vi "Get Job Data.vi"(0 "SystemLink repo in":T3, 5 "job ID":string, 11 "error in (no error)":errorcluster) -> (4 "SystemLink repo out":T3, 6 "job data":T1, 15 "error out":errorcluster)   [LabVIEW 2017, in "SystemLink_Repo_API.lvlib"]
doc: "Returns the job data for the specified job ID."
uses:
  SystemLink_Repo_API.lvlib
  systemlink repo.ctl
  <vilib>/httpClient/ClientHandle.ctl
  syslink_job.ctl
  syslink_job_datatype.ctl
  <vilib>/httpClient/LabVIEWHTTPClient.lvlib
panel:
  out "body":string
  out "headers":string
  # "Status will be \"SUCCEEDED\" for a successful job and \"FAILED\" for a failed job."
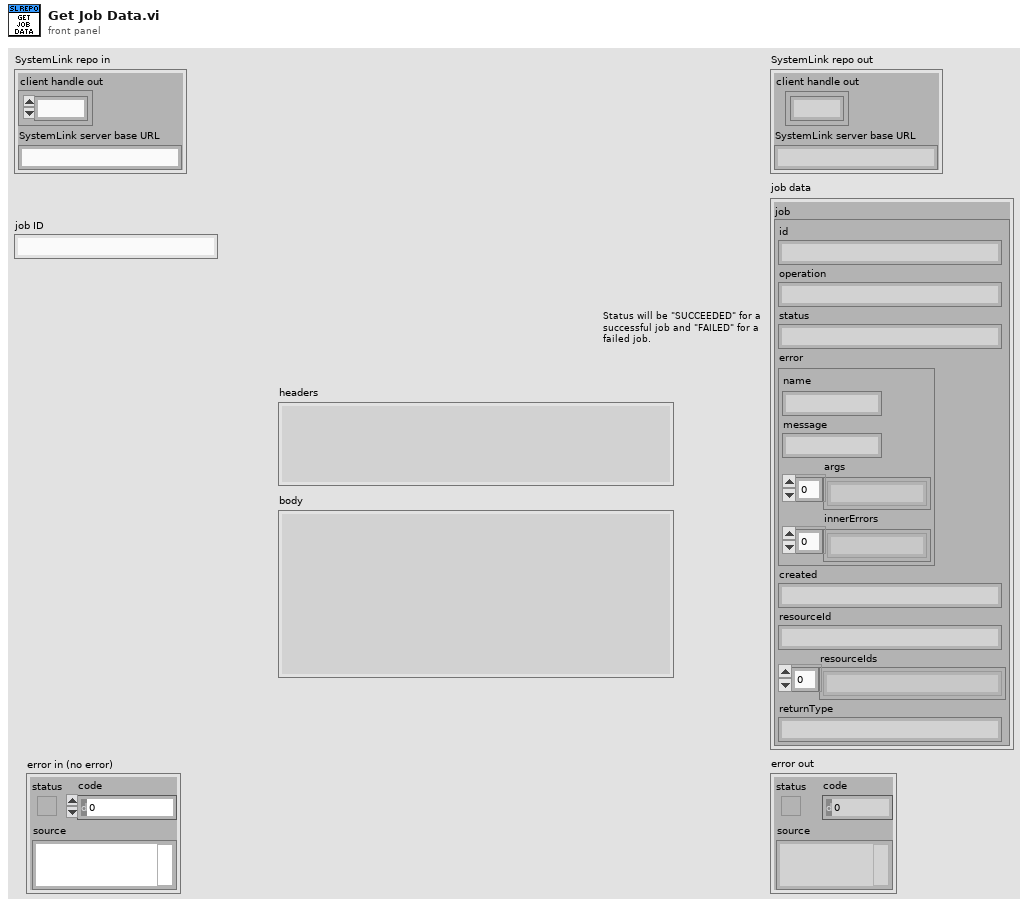
[diagram p1: front panel]
types:
  T1 = typedef "SystemLink_Repo_API.lvlib/syslink_job.ctl" = cluster{"job":T2}
  T2 = typedef "SystemLink_Repo_API.lvlib/syslink_job_datatype.ctl" = cluster{"id":string, "operation":string, "status":string, "error":cluster{"name":string, "message":string, "args":string[], "innerErrors":string[]}, "created":string, "resourceId":string, "resourceIds":string[], "returnType":string}
  T3 = typedef "SystemLink_Repo_API.lvlib/systemlink repo.ctl" = cluster{"client handle out":T4, "SystemLink server base URL":string}
  T4 = typedef "LabVIEWHTTPClient.lvlib/ClientHandle.ctl" = refnum<k1>
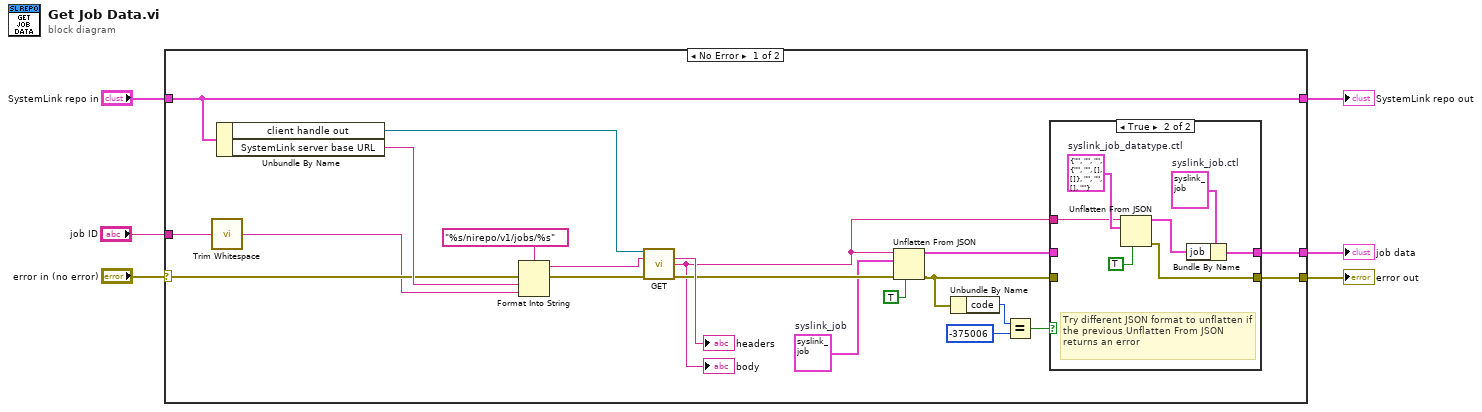
[diagram p0: block diagram]
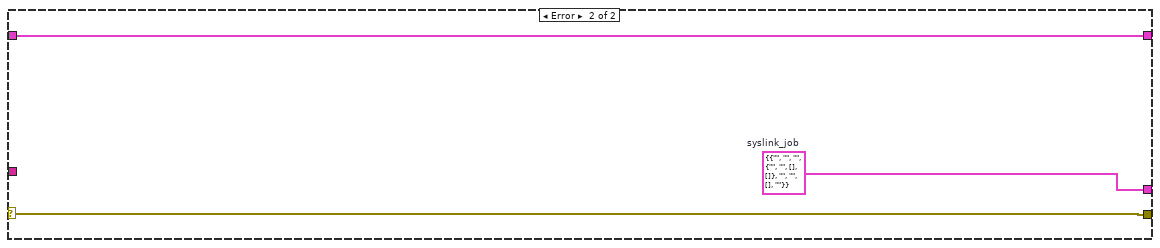
[diagram p3: hidden frame]
diagram:
  n1 = case shown="No Error" "error in (no error)" {
    selector: "error in (no error)" -> [w22 w39]
    tunnel: "SystemLink repo in" -> [w15 w37]
    tunnel: [w8 w39] -> w5
    tunnel: "job ID" -> [w17 _]
    tunnel: [w10 w38] -> w3
    tunnel: [w15 w37] -> w1
    frame No Error {
      w16 = T1 {"job"={"id"="", "operation"="", "status"="", "error"={"name"="", "message"="", "args"=[], "innerErrors"=[]}, "created"="", "resourceId"="", "resourceIds"=[], "returnType"=""}}  # syslink_job
      n2 = call <vilib>:"Trim Whitespace.vi"("string"=w17) -> ("trimmed string"=w18:string)  [unwired: 1 in]
      n3 = Unbundle By Name(w15) -> ("client handle out"=w24:T4, "SystemLink server base URL"=w23:string)
      n4 = Format Into String(format string="%s/nirepo/v1/jobs/%s", error in=w22, w23, w18) -> (resulting string=w25:string, error out=w21:errorcluster)  [unwired: 1 in]
      n5 = call <vilib>:"GET.vi"("client handle"=w24, "url"=w25, "error in (no error)"=w21) -> ("headers"=→"headers":string, "body"=w7:string, "error out"=w19:errorcluster)  [unwired: 9 in, 1 out]
      "body" <- w7
      n6 = Unflatten From JSON(JSON string=w7, type and defaults=w16, default null elements? (F)=TRUE, error in (no error)=w19) -> (value=w11:T1, error out=w9:errorcluster)  [unwired: 3 in]
      n7 = Unbundle By Name(w9) -> ("code"=w14:i32)
      n8 = Equal?(x=w14, y=-375006) -> (x = y?=w12:bool)
      n9 = case shown="True" w12 {
        tunnel: w11 -> [w29 _]
        tunnel: [w29 w32] -> w10
        tunnel: w9 -> [w28 _]
        tunnel: [w28 w30] -> w8
        tunnel: w7 -> [_ w35]
        frame False {
        }
        frame True {
          w34 = T1 {"job"={"id"="", "operation"="", "status"="", "error"={"name"="", "message"="", "args"=[], "innerErrors"=[]}, "created"="", "resourceId"="", "resourceIds"=[], "returnType"=""}}  # syslink_job.ctl
          w36 = T2 {"id"="", "operation"="", "status"="", "error"={"name"="", "message"="", "args"=[], "innerErrors"=[]}, "created"="", "resourceId"="", "resourceIds"=[], "returnType"=""}  # syslink_job_datatype.ctl
          # "Try different JSON format to unflatten if the previous Unflatten From JSON returns an error"
          n10 = Unflatten From JSON(JSON string=w35, type and defaults=w36, default null elements? (F)=TRUE) -> (value=w33:T2, error out=w30:errorcluster)  [unwired: 4 in]
          n11 = Bundle By Name(cluster=w34, "job"=w33) -> (w32:T1)
        }
      }
    }
    frame Error {
      w38 = T1 {"job"={"id"="", "operation"="", "status"="", "error"={"name"="", "message"="", "args"=[], "innerErrors"=[]}, "created"="", "resourceId"="", "resourceIds"=[], "returnType"=""}}  # syslink_job
    }
  }
  "error out" <- w5
  "SystemLink repo out" <- w1
  "job data" <- w3
